vi "system status.vi"() -> ()   [LabVIEW 2016]
panel:
  out "System Status":string
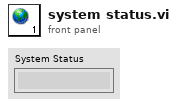
[diagram p1: front panel]
diagram:
